vi "Linear Interpolation GPM to Percent Open.vi"(9 "Interp Direction":enum16{"GPM to Percent", "Percent to GPM"}(ring), 10 "Input (GPM,Percent)":dbl, 11 "Configuration":T1=enum."Global, Tank") -> (2 "Output (Percent,GPM)":dbl)   [LabVIEW 2012]
uses:
  TestedFlowratesScenarios.ctl
  Global HEWH.vi
  <vilib>/gmath/NI_Gmath.lvlib
panel:
  # "Measured in test lab."
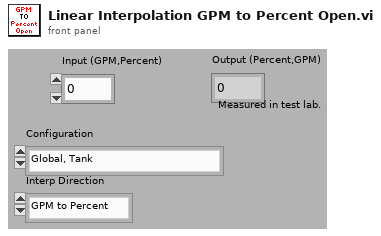
[diagram p1: front panel]
types:
  T1 = typedef "TestedFlowratesScenarios.ctl" = enum16{"DRK500,Station1", "DRK375,Lab", "SRK500,Station1,5GPM FR", "DRK375,STATION3,1/2\"HOSE", "DRK500,Station1,downspout", "DRK375,Station3,thruEcocute", "DRK375,Station3,purge", "Build2,2B,Purge", "Global, Purge", "Global, Tank"}
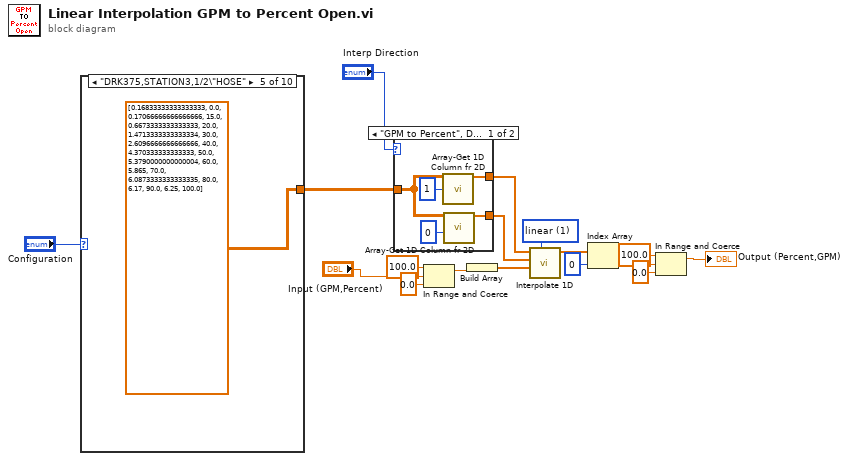
[diagram p0: block diagram]
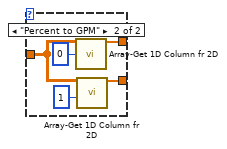
[diagram p2: hidden frame]
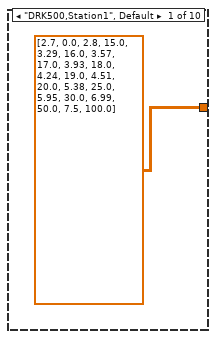
[diagram p3: hidden frame]
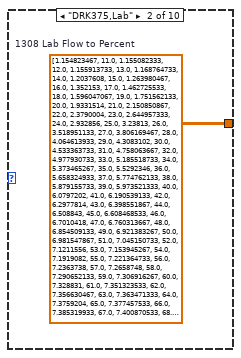
[diagram p4: hidden frame]
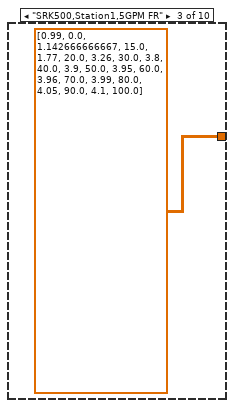
[diagram p5: hidden frame]
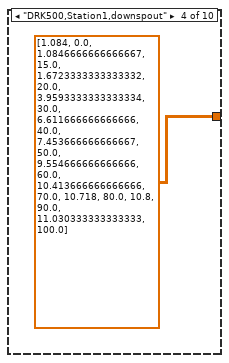
[diagram p6: hidden frame]
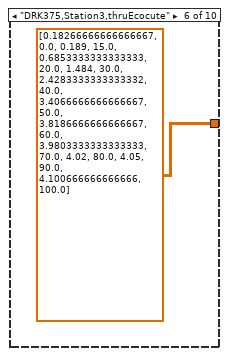
[diagram p7: hidden frame]
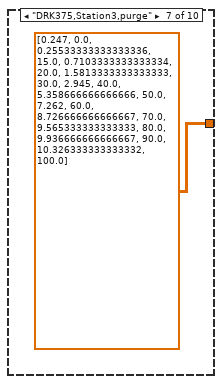
[diagram p8: hidden frame]
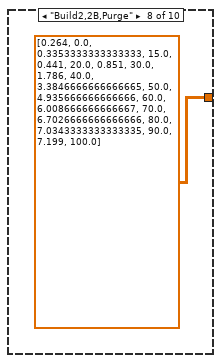
[diagram p9: hidden frame]
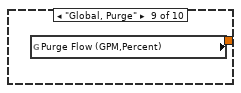
[diagram p10: hidden frame]
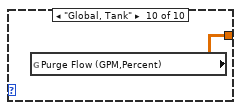
[diagram p11: hidden frame]
diagram:
  w17 = 1 items=["nearest", "linear", "spline", "cubic Hermite", "Lagrange"] ("method")
  n1 = case shown="\"DRK375,STATION3,1/2\\\"HOSE\"" "Configuration" {
    tunnel: [dbl[][] [[2.7, 0.0], [2.8, 15.0], [3.29, 16.0], [3.57, 17.0], [3.93, 18.0], [4.24, 19.0], [4.51, 20.0], [5.38, 25.0], [5.95, 30.0], [6.99, 50.0], [7.5, 100.0]] ("DRK500 thru Small Flowmeter") w19 dbl[][] [[0.99, 0.0], [1.142666666667, 15.0], [1.77, 20.0], [3.26, 30.0], [3.8, 40.0], [3.9, 50.0], [3.95, 60.0], [3.96, 70.0], [3.99, 80.0], [4.05, 90.0], [4.1, 100.0]] ("transposed array") dbl[][] [[1.084, 0.0], [1.0846666666666667, 15.0], [1.6723333333333332, 20.0], [3.9593333333333334, 30.0], [6.611666666666666, 40.0], [7.453666666666667, 50.0], [9.554666666666666, 60.0], [10.413666666666666, 70.0], [10.718, 80.0], [10.8, 90.0], [11.030333333333333, 100.0]] ("Results(Flow,Percent)") dbl[][] [[0.16833333333333333, 0.0], [0.17066666666666666, 15.0], [0.6673333333333333, 20.0], [1.4713333333333334, 30.0], [2.6096666666666666, 40.0], [4.370333333333333, 50.0], [5.3790000000000004, 60.0], [5.865, 70.0], [6.0873333333333335, 80.0], [6.17, 90.0], [6.25, 100.0]] ("Results(Flow,Percent)") dbl[][] [[0.18266666666666667, 0.0], [0.189, 15.0], [0.6853333333333333, 20.0], [1.484, 30.0], [2.4283333333333332, 40.0], [3.4066666666666667, 50.0], [3.8186666666666667, 60.0], [3.9803333333333333, 70.0], [4.02, 80.0], [4.05, 90.0], [4.100666666666666, 100.0]] ("Results(Flow,Percent)") dbl[][] [[0.247, 0.0], [0.25533333333333336, 15.0], [0.7103333333333334, 20.0], [1.5813333333333333, 30.0], [2.945, 40.0], [5.358666666666666, 50.0], [7.262, 60.0], [8.726666666666667, 70.0], [9.565333333333333, 80.0], [9.936666666666667, 90.0], [10.326333333333332, 100.0]] ("Results(Flow,Percent)") dbl[][] [[0.264, 0.0], [0.3353333333333333, 15.0], [0.441, 20.0], [0.851, 30.0], [1.786, 40.0], [3.3846666666666665, 50.0], [4.935666666666666, 60.0], [6.008666666666667, 70.0], [6.7026666666666666, 80.0], [7.0343333333333335, 90.0], [7.199, 100.0]] ("Results(Flow,Percent)") w26 w27] -> w7
    frame "DRK500,Station1", Default {
    }
    frame "DRK375,Lab" {
      w19 = dbl[][] [[1.154823467, 11.0], [1.155082333, 12.0], [1.155913733, 13.0], [1.168764733, 14.0], [1.2037608, 15.0], [1.263980467, 16.0], [1.352153, 17.0], [1.462725533, 18.0], [1.596047067, 19.0], [1.751562133, 20.0], [1.9331514, 21.0], [2.150850867, 22.0], [2.3790004, 23.0], [2.644957333, 24.0], [2.932856, 25.0], [3.23813, 26.0], [3.518951133, 27.0], [3.806169467, 28.0], [4.064613933, 29.0], [4.3083102, 30.0], [4.533363733, 31.0], [4.758063667, 32.0], [4.977930733, 33.0], [5.185518733, 34.0], [5.373465267, 35.0], [5.5292346, 36.0], [5.658324933, 37.0], [5.774762133, 38.0], [5.879155733, 39.0], [5.973521333, 40.0], [6.0797202, 41.0], [6.190539133, 42.0], [6.2977814, 43.0], [6.398551867, 44.0], [6.508843, 45.0], [6.608468533, 46.0], [6.7010418, 47.0], [6.760313667, 48.0], [6.854509133, 49.0], [6.921383267, 50.0], [6.981547867, 51.0], [7.045150733, 52.0], [7.1211556, 53.0], [7.153945267, 54.0], [7.1919082, 55.0], [7.221364733, 56.0], [7.2363738, 57.0], [7.2658748, 58.0], [7.290652133, 59.0], [7.306916267, 60.0], [7.328831, 61.0], [7.351323533, 62.0], [7.356630467, 63.0], [7.363471333, 64.0], [7.3759204, 65.0], [7.377457533, 66.0], [7.385319933, 67.0], [7.400870533, 68.0], [7.420039867, 69.0], [7.436503867, 70.0], [7.435100667, 71.0], [7.441507067, 72.0], [7.4586758, 73.0], [7.4709312, 74.0], [7.477849933, 75.0], [7.502882667, 76.0], [7.515599867, 77.0], [7.516479467, 78.0], [7.5161762, 79.0], [7.522149933, 80.0], [7.531457467, 81.0], [7.540166067, 82.0], [7.545417133, 83.0], [7.547076867, 84.0], [7.544551533, 85.0], [7.527355067, 86.0], [7.531499133, 87.0], [7.540953933, 88.0], [7.553015733, 89.0], [7.5680518, 90.0], [7.595900467, 91.0], [7.600769333, 92.0], [7.603110267, 93.0], [7.608227533, 94.0], [7.615357067, 95.0], [7.613050067, 96.0], [7.632628733, 97.0], [7.6430432, 98.0]]  # 1308 Lab Flow to Percent
    }
    frame "SRK500,Station1,5GPM FR" {
    }
    frame "DRK500,Station1,downspout" {
    }
    frame "DRK375,STATION3,1/2\"HOSE" {
    }
    frame "DRK375,Station3,thruEcocute" {
    }
    frame "DRK375,Station3,purge" {
    }
    frame "Build2,2B,Purge" {
    }
    frame "Global, Purge" {
      n2 = global read "Global HEWH.vi" "Purge Flow (GPM,Percent)"() -> (w26:dbl[][])
    }
    frame "Global, Tank" {
      n3 = global read "Global HEWH.vi" "Purge Flow (GPM,Percent)"() -> (w27:dbl[][])
    }
  }
  n4 = case shown="\"GPM to Percent\", Default" "Interp Direction" {
    tunnel: [w30 w35] -> w13
    tunnel: [w29 w34] -> w12
    tunnel: w7 -> [w28 w33]
    frame "GPM to Percent", Default {
      n5 = call "Array-Get 1D Column fr 2D.vi"("2D Array Data"=w28, "column index"=1) -> ("Column Data"=w29:dbl[])  [unwired: 13 in]
      n6 = call "Array-Get 1D Column fr 2D.vi"("2D Array Data"=w28, "column index"=0) -> ("Column Data"=w30:dbl[])  [unwired: 13 in]
    }
    frame "Percent to GPM" {
      n7 = call "Array-Get 1D Column fr 2D.vi"("2D Array Data"=w33, "column index"=0) -> ("Column Data"=w34:dbl[])  [unwired: 13 in]
      n8 = call "Array-Get 1D Column fr 2D.vi"("2D Array Data"=w33, "column index"=1) -> ("Column Data"=w35:dbl[])  [unwired: 13 in]
    }
  }
  n9 = In Range and Coerce(upper limit=100.0, x="Input (GPM,Percent)", lower limit=0.0) -> (coerced(x)=w1:dbl)  [unwired: 1 out]
  n10 = Build Array(w1) -> (w16:dbl[])
  n11 = call <vilib>:"Interpolate 1D.vi"("method"=w17, "xi"=w16, "X"=w13, "Y"=w12) -> ("yi"=w15:dbl[])  [unwired: 5 in, 2 out]
  n12 = Index Array(array=w15, index=0) -> (element=w11:dbl)
  n13 = In Range and Coerce(upper limit=100.0, x=w11, lower limit=0.0) -> (coerced(x)=→"Output (Percent,GPM)":dbl)  [unwired: 1 out]
